vi "encodeInt8.vi"(2 "Compress? (T)":bool=TRUE, 3 "Int8":i8) -> (1 "MessagePack":u8[](array[numeric]) format="%.0x")   [LabVIEW 2015, in "MsgPack.lvlib"]
uses:
  MsgPack.lvlib
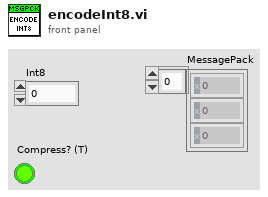
[diagram p1: front panel]
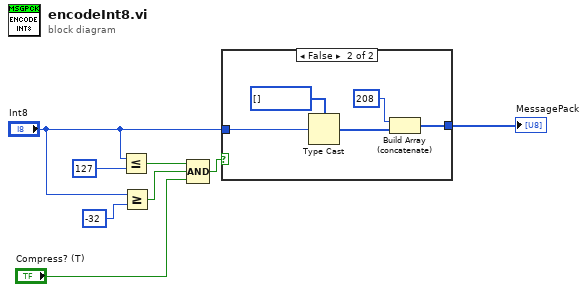
[diagram p0: block diagram]
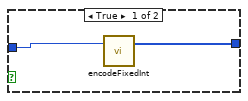
[diagram p2: hidden frame]
diagram:
  n1 = Less Or Equal?(x="Int8", y=i8 127) -> (x <= y?=w5:bool)
  n2 = Greater Or Equal?(x="Int8", y=i8 -32) -> (x >= y?=w4:bool)
  n3 = Compound Arithmetic op=AND(w5, w4, "Compress? (T)") -> (w2:bool)
  n4 = case shown="False" w2 {
    tunnel: [w10 w15] -> w8
    tunnel: "Int8" -> [w9 w11]
    frame True {
      n5 = call "encodeFixedInt.vi"("FixedInt8"=w9) -> ("Array"=w10:u8[])  [unwired: 2 in]
    }
    frame False {
      n6 = Type Cast(type=u8[] [], x=w11) -> (*(type *) &x=w12:u8[])
      n7 = Build Array (concatenate)(u8 208, w12) -> (w15:u8[])
    }
  }
  "MessagePack" <- w8
